vi "HAPS_LoadTable_SetBeam_Auto.vi"() -> ()   [LabVIEW 2023, in "HAPS.lvlib"]
uses:
  HAPS.lvlib
  set_ele.ctl
  <vilib>/Utility/file.llb/Read Delimited Spreadsheet (string).vi
  HAPS_MCU_ELE_Func.ctl
panel:
  out "Remaining Files":i32
  out "Remaining quantity":i32
  out "Table_FileName":path
  in  "file path (dialog if empty)":path
  out "ele phase":i32
  out "ele gain":i32
  out "channel":i32
  out "chain ID":i32
  out "group":i32
  out "array id":i32
  # "HAPS 4pcs * 24x24 In Phase Setting"
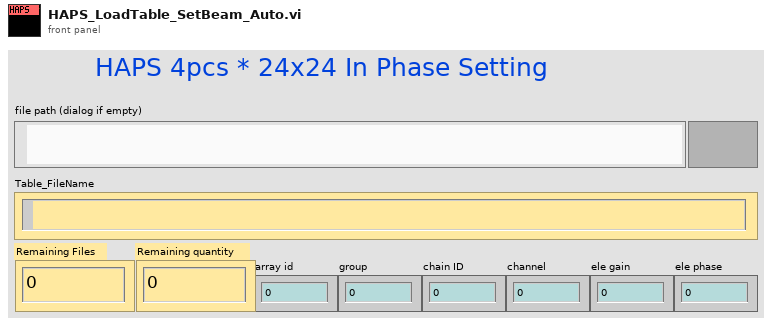
[diagram p1: front panel]
types:
  T1 = typedef "HAPS.lvlib/set_ele.ctl" = cluster{"ch":i32, "chain_id":i32, "group":i32, "array_id":i32, "ele_phase":i32, "ele_gain":i32, "com_gain":i32, "pd_range":i32}
  T2 = typedef "HAPS.lvlib/HAPS_MCU_ELE_Func.ctl" = enum16{"array_init", "set_com_gain", "set_ch_gain_phase", "set_pd_range", "get_preamp_temp", "get_bfic_temp", "get_tx_pd", "ch_on", "ch_ctrl_all", "array_ctrl_src"}
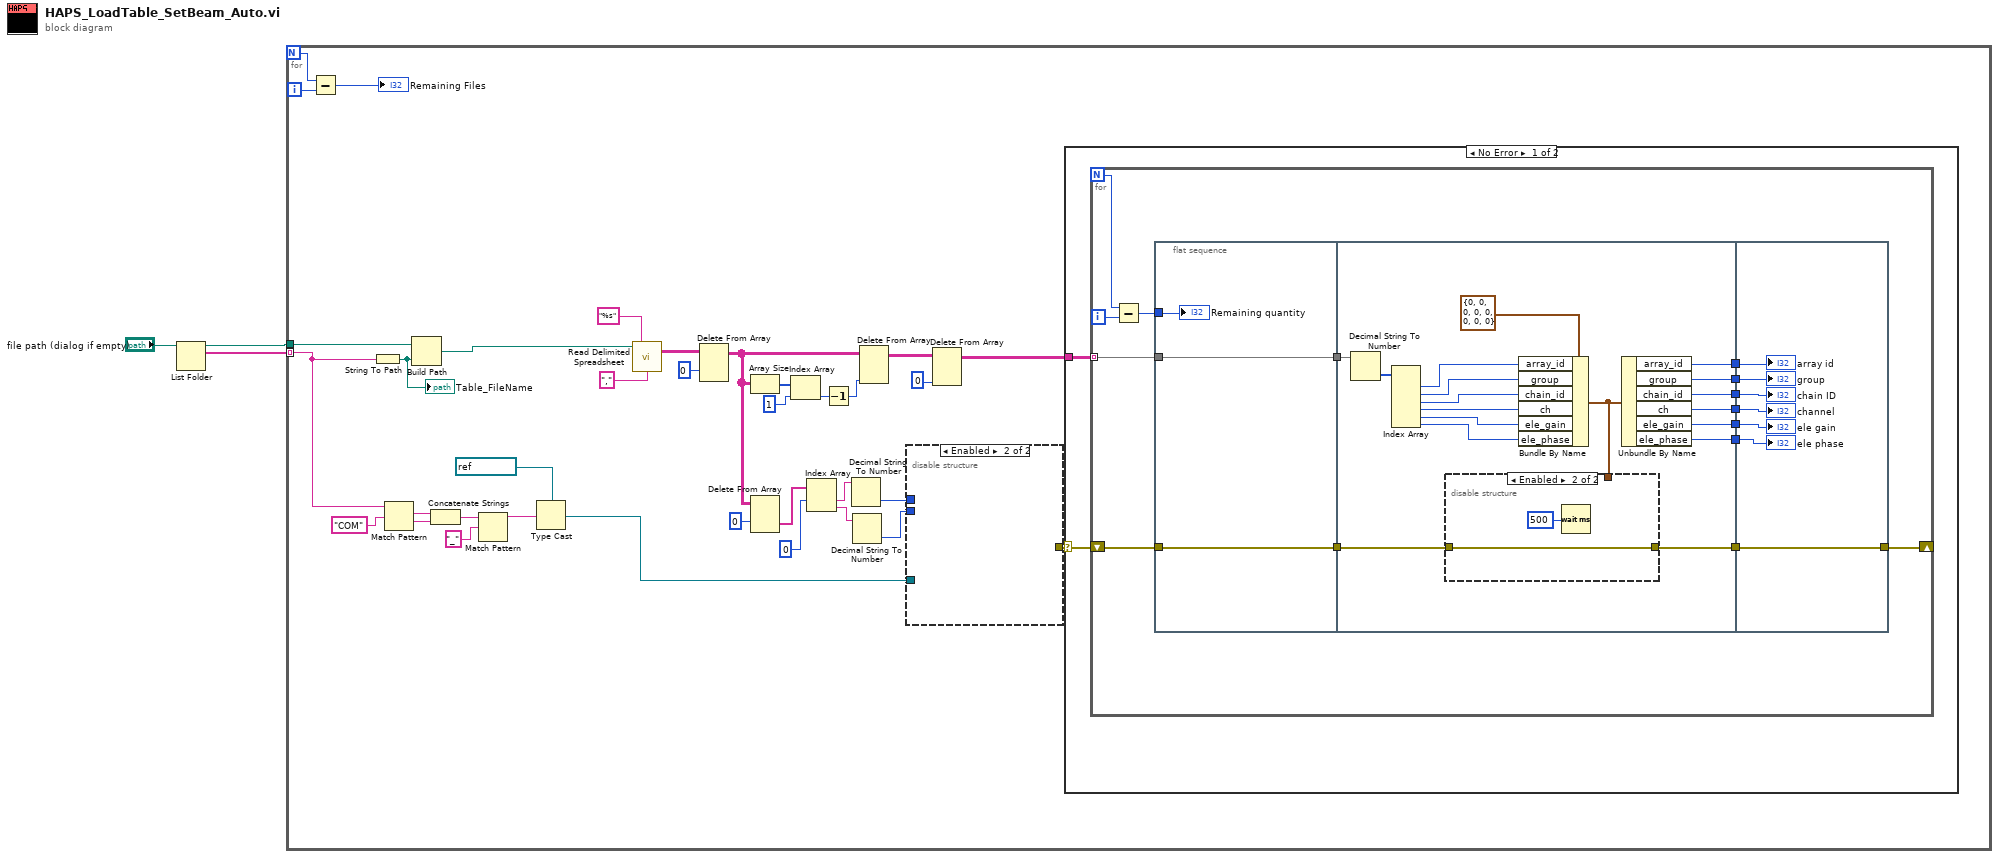
[diagram p0: block diagram]
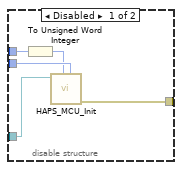
[diagram p2: hidden frame]
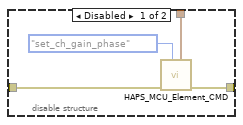
[diagram p3: hidden frame]
diagram:
  n1 = List Folder(path="file path (dialog if empty)") -> (path out=w2:path, filenames=w1:string[])  [unwired: 3 in, 2 out]
  n2 = for {
    N -> [w6]
    tunnel: w2 -> [w18]
    tunnel: w1 -> [w16] mode=indexing
    i -> [w5]
    n3 = Subtract(x=w6, y=w5) -> (x-y=→"Remaining Files":i32)
    n4 = String To Path(string=w16) -> (path=w17:path)
    "Table_FileName" <- w17
    n5 = Match Pattern(string=w16, regular expression="COM") -> (match substring=w10:string, after substring=w13:string)  [unwired: 1 in, 2 out]
    n6 = Build Path(base path=w18, name or relative path=w17) -> (appended path=w15:path)
    n7 = Concatenate Strings(w10, w13) -> (w11:string)
    n8 = Match Pattern(string=w11, regular expression="_") -> (before substring=w9:string)  [unwired: 1 in, 3 out]
    n9 = Type Cast(type=refnum<visa-resource-name> "COM1" ("VISA resource name"), x=w9) -> (*(type *) &x=w7:refnum<visa-resource-name>)
    n10 = call-poly <vilib>:"Read Delimited Spreadsheet.vi"("file path (dialog if empty)"=w15, "format (%s)"="%s" ("format (%.3f)"), "delimiter (\\t)"="," ("delimiter (\\t)")) -> ("all rows"=w36:string[][])  [unwired: 7 in, 5 out]
    n11 = Delete From Array(array=w36, index (row)=0) -> (array with subset deleted=w25:string[][])  [unwired: 2 in, 1 out]
    n12 = Array Size(array=w25) -> (size(s)=w34:i32[])
    n13 = Delete From Array(array=w25, index (row)=0) -> (deleted portion=w24:string[])  [unwired: 2 in, 1 out]
    n14 = Index Array(array=w34, index=1) -> (element=w31:i32)
    n15 = Index Array(array=w24, index #1=0 ("index")) -> (element #1=w23:string, element #2=w22:string)  [unwired: 1 in]
    n16 = Decrement(x=w31) -> (x-1=w33:i32)
    n17 = Decimal String To Number(string=w23) -> (number=w20:i32)  [unwired: 2 in, 1 out]
    n18 = Decimal String To Number(string=w22) -> (number=w19:i32)  [unwired: 2 in, 1 out]
    n19 = Delete From Array(array=w25, index (col)=w33) -> (array with subset deleted=w29:string[][])  [unwired: 2 in, 1 out]
    n20 = disable-structure shown="Enabled" {
      disable-tunnel: [w43 _] -> w30
      disable-tunnel: w20 -> [w42 _]
      disable-tunnel: w19 -> [w41 _]
      disable-tunnel: w7 -> [w40 _]
      frame Disabled {
        n21 = To Unsigned Word Integer(number=w42) -> (unsigned 16bit integer=w39:u16)
        n22 = call "HAPS_MCU_Init.vi"("array_id"=w41, "Tx/Rx"=w39, "VISA resource name"=w40) -> ("error out"=w43:errorcluster)  [unwired: 8 in]
      }
      frame Enabled {
      }
    }
    n23 = Delete From Array(array=w29, index (col)=0 ("index (row)")) -> (array with subset deleted=w28:string[][])  [unwired: 2 in, 1 out]
    n24 = case shown="No Error" w30 {
      selector: w30 -> [w44 _]
      tunnel: w28 -> [w45 _]
      frame No Error {
        n25 = for {
          N -> [w54]
          tunnel: w45 -> [w60] mode=indexing
          shift-right: [w59] -> _
          shift-left: w44 -> [w58]
          i -> [w55]
          n26 = Subtract(x=w54, y=w55) -> (x-y=w53:i32)
          n27 = flat-sequence {
            tunnel: w58 -> [w62]
            tunnel: w60 -> [w63]
            tunnel: [w63] -> w57
            tunnel: [w62] -> w56
            tunnel: w53 -> [w61]
            tunnel: w57 -> [w81]
            tunnel: w56 -> [w78]
            tunnel: [w79] -> w52
            tunnel: [w69] -> w51
            tunnel: [w68] -> w50
            tunnel: [w67] -> w49
            tunnel: [w66] -> w48
            tunnel: [w65] -> w47
            tunnel: [w64] -> w46
            tunnel: [w94] -> w59
            tunnel: w52 -> [w94]
            tunnel: w51 -> [w93]
            tunnel: w50 -> [w92]
            tunnel: w49 -> [w91]
            tunnel: w48 -> [w90]
            tunnel: w47 -> [w89]
            tunnel: w46 -> [w88]
            frame #0 {
              "Remaining quantity" <- w61
            }
            frame #1 {
              n28 = Decimal String To Number(string=w81) -> (number=w80:i32[])  [unwired: 2 in, 1 out]
              n29 = Index Array(array=w80) -> (element #1=w76:i32, element #2=w75:i32, element #3=w74:i32, element #4=w73:i32, element #5=w72:i32, element #6=w71:i32)  [unwired: 6 in]
              n30 = Bundle By Name(cluster=T1 {"ch"=0, "chain_id"=0, "group"=0, "array_id"=0, "ele_phase"=0, "ele_gain"=0, "com_gain"=0, "pd_range"=0} ("set_ele"), "array_id"=w76, "group"=w75, "chain_id"=w74, "ch"=w73, "ele_gain"=w72, "ele_phase"=w71) -> (w70:T1)
              n31 = disable-structure shown="Enabled" {
                disable-tunnel: [w85 w87] -> w79
                disable-tunnel: w78 -> [w84 w87]
                disable-tunnel: w70 -> [w82 _]
                frame Disabled {
                  n32 = call "HAPS_MCU_Element_CMD.vi"("set_ele"=w82, "HAPS_MCU_ELE_Func."=HAPS_MCU_ELE_Func."set_ch_gain_phase", "error in"=w84) -> ("error out"=w85:errorcluster)  [unwired: 7 in, 1 out]
                }
                frame Enabled {
                  n33 = Wait (ms)(milliseconds to wait=u32 500) -> ()  [unwired: 1 out]
                }
              }
              n34 = Unbundle By Name(w70) -> ("array_id"=w69:i32, "group"=w68:i32, "chain_id"=w67:i32, "ch"=w66:i32, "ele_gain"=w65:i32, "ele_phase"=w64:i32)
            }
            frame #2 {
              "group" <- w92
              "chain ID" <- w91
              "channel" <- w90
              "ele gain" <- w89
              "ele phase" <- w88
              "array id" <- w93
            }
          }
        }
      }
      frame Error {
      }
    }
  }
